vi "SAOMM-OFFSET.vi"(0 "Hexapod VRN":refnum<visa-resource-name>="COM4", 1 "Active Refnum":refnum<vi>, 2 "PrAMS-ACK":refnum<vi>, 7 "output cluster":T1, 13 "MessageType":cluster{string[], u32[]}={["emtError", "emtAreYouThere", "emtAcknowledgment", "emtGetClientType", "emtClientType", "emtGetImageExposureTime", "emtSetImageExposureTime", "emtImageExposureTime", "emtGetOptimalExposureTime", "emtSetOptimalExposureTime", "emtOptimalExposureTime", "emtGetImageEMGain", "emtSetImageEMGain", "emtImageEMGain", "emtGetFPGACtrl", "emtSetFPGACtrl", "emtFPGACtrl", "emtGetImageWidth", "emtSetImageWidth", "emtImageWidth", "emtGetImageHeight", "emtSetImageHeight", "emtImageHeight", "emtGetImageBinning", "emtSetImageBinning", "emtImageBinning", "emtGetImageDisplayFrameRate", "emtSetImageDisplayFrameRate", "emtImageDisplayFrameRate", "emtGetROIWidth", "emtSetROIWidth", "emtROIWidth", "emtGetROIHeight", "emtSetROIHeight", "emtROIHeight", "emtGetROIXOffset", "emtSetROIXOffset", "emtROIXOffset", "emtGetROIYOffset", "emtSetROIYOffset", "emtROIYOffset", "emtStartAcquisition", "mtStopAcquisition", "emtAcquisitionStarted", "emtAcquisitionStopped", "emtGetFalconImage", "emtFalconImage"], [1, 2, 3, 4, 5, 1001, 1101, 1201, 1002, 1102, 1202, 1003, 1103, 1203, 1004, 1104, 1204, 1005, 1105, 1205, 1006, 1106, 1206, 1007, 1107, 1207, 1008, 1108, 1208, 1009, 1109, 1209, 1010, 1110, 1210, 1011, 1111, 1211, 1012, 1112, 1212, 1130, 1131, 1150, 1151, 1070, 1270]}) -> (8 "Error":bool)   [LabVIEW 2019]
uses:
  Polymorphics/Num2littleEndian(DBL).vi
panel:
  out "First Run":bool
  in  "Signature":u32=1886544237
  in  "X":dbl caption="Pos" min=-5.0 max=5.0 format="%.4f"
  in  "Y":dbl caption="Pos" min=-5.0 max=5.0 format="%.4f"
  in  "Z":dbl caption="Pos" min=-5.0 max=5.0 format="%.4f"
  in  "U":dbl caption="Pos" min=-1.0 max=1.0 format="%.4f"
  in  "V":dbl caption="Pos" min=-1.0 max=1.0 format="%.4f"
  # "DÉPLACEMENTS"
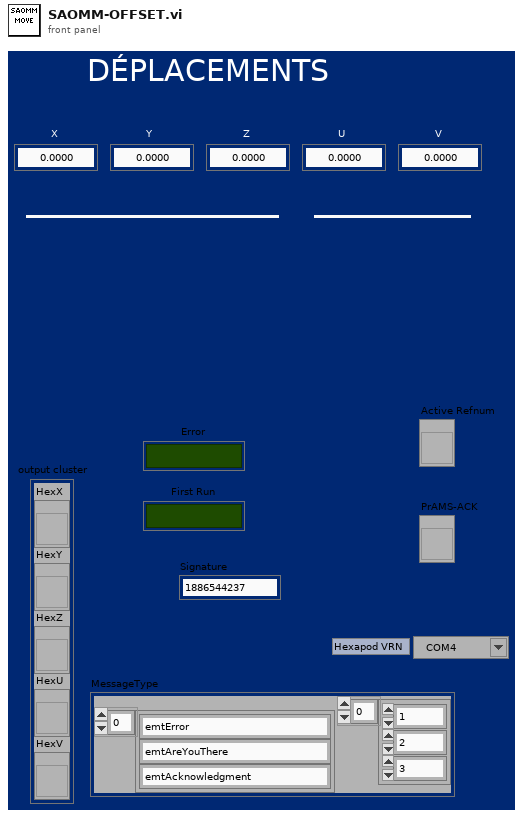
[diagram p1: front panel]
types:
  T1 = cluster{"HexX":refnum<vi>, "HexY":refnum<vi>, "HexZ":refnum<vi>, "HexU":refnum<vi>, "HexV":refnum<vi>}
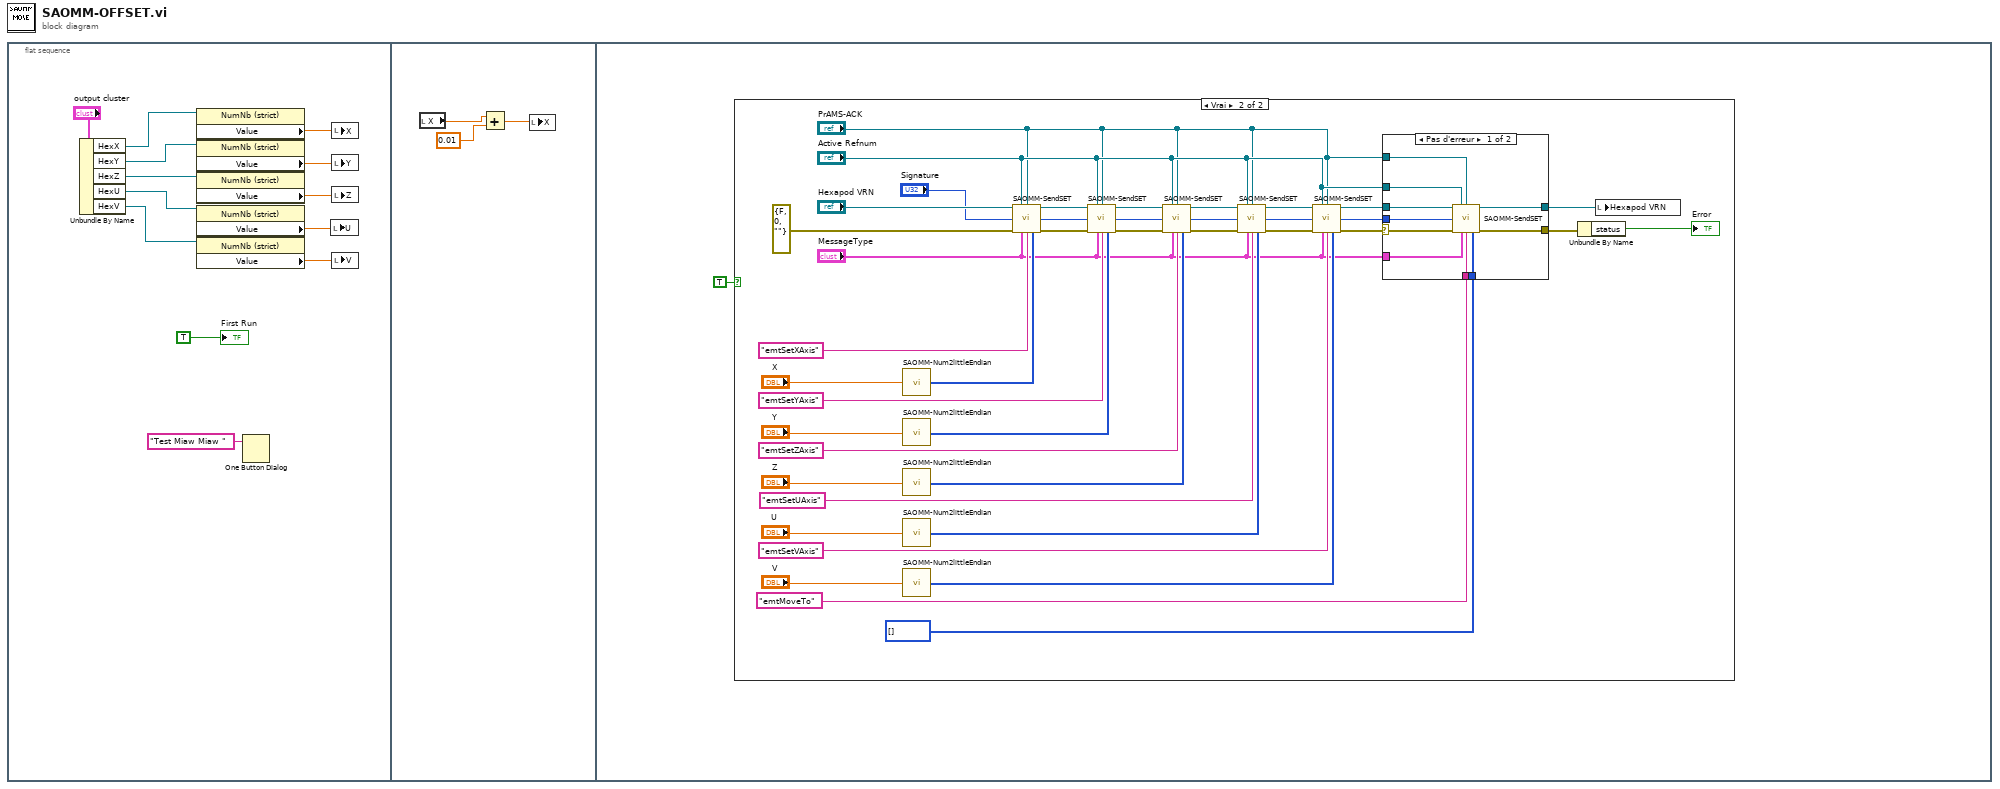
[diagram p0: block diagram]
diagram:
  n1 = flat-sequence {
    frame #0 {
      n2 = Unbundle By Name("output cluster") -> ("HexX"=w11:refnum<vi>, "HexY"=w10:refnum<vi>, "HexZ"=w9:refnum<vi>, "HexU"=w8:refnum<vi>, "HexV"=w7:refnum<vi>)
      n3 = property class="NumNb (strict)"(reference=w11) -> ("Value"=w2:dbl)  [unwired: 1 in, 2 out]
      n4 = property class="NumNb (strict)"(reference=w10) -> ("Value"=w3:dbl)  [unwired: 1 in, 2 out]
      n5 = property class="NumNb (strict)"(reference=w9) -> ("Value"=w4:dbl)  [unwired: 1 in, 2 out]
      n6 = property class="NumNb (strict)"(reference=w8) -> ("Value"=w5:dbl)  [unwired: 1 in, 2 out]
      n7 = property class="NumNb (strict)"(reference=w7) -> ("Value"=w6:dbl)  [unwired: 1 in, 2 out]
      n8 = One Button Dialog(message="Test Miaw Miaw ") -> ()  [unwired: 1 in, 1 out]
      n9 = local write "U"(w5) -> ()
      n10 = local write "X"(w2) -> ()
      n11 = local write "Y"(w3) -> ()
      n12 = local write "Z"(w4) -> ()
      n13 = local write "V"(w6) -> ()
      "First Run" <- TRUE
    }
    frame #1 {
      n14 = local read "X"() -> (w15:dbl)
      n15 = Add(x=w15, y=0.01) -> (x+y=w16:dbl)
      n16 = local write "X"(w16) -> ()
    }
    frame #2 {
      n17 = case shown="Vrai" TRUE {
        frame False {
        }
        frame True {
          n18 = call-poly "SAOMM-Num2littleEndian.vi"("Number"="X") -> ("LiitleEndianedData"=w40:u8[])  [unwired: 14 in]
          n19 = call-poly "SAOMM-Num2littleEndian.vi"("Number"="Y") -> ("LiitleEndianedData"=w41:u8[])  [unwired: 14 in]
          n20 = call-poly "SAOMM-Num2littleEndian.vi"("Number"="Z") -> ("LiitleEndianedData"=w42:u8[])  [unwired: 14 in]
          n21 = call-poly "SAOMM-Num2littleEndian.vi"("Number"="U") -> ("LiitleEndianedData"=w45:u8[])  [unwired: 14 in]
          n22 = call-poly "SAOMM-Num2littleEndian.vi"("Number"="V") -> ("LiitleEndianedData"=w46:u8[])  [unwired: 14 in]
          n23 = call "SAOMM-SendSET.vi"("PRAMMS-COMM IN"="Hexapod VRN", "Active Refnum"="Active Refnum", "PrAMS-ACK"="PrAMS-ACK", "Signature"="Signature", "Error IN"=errorcluster {"status"=FALSE, "code"=0, "source"=""}, "MessageType"="MessageType", "Active SET"="emtSetXAxis", "Value (little endianed byte array)"=w40) -> ("PRAMMS-COMM OUT"=w31:refnum<visa-resource-name>, "Error OUT"=w37:errorcluster)  [unwired: 4 in, 2 out]
          n24 = call "SAOMM-SendSET.vi"("PRAMMS-COMM IN"=w31, "Active Refnum"="Active Refnum", "PrAMS-ACK"="PrAMS-ACK", "Signature"="Signature", "Error IN"=w37, "MessageType"="MessageType", "Active SET"="emtSetYAxis", "Value (little endianed byte array)"=w41) -> ("PRAMMS-COMM OUT"=w32:refnum<visa-resource-name>, "Error OUT"=w36:errorcluster)  [unwired: 4 in, 2 out]
          n25 = call "SAOMM-SendSET.vi"("PRAMMS-COMM IN"=w32, "Active Refnum"="Active Refnum", "PrAMS-ACK"="PrAMS-ACK", "Signature"="Signature", "Error IN"=w36, "MessageType"="MessageType", "Active SET"="emtSetZAxis", "Value (little endianed byte array)"=w42) -> ("PRAMMS-COMM OUT"=w52:refnum<visa-resource-name>, "Error OUT"=w35:errorcluster)  [unwired: 4 in, 2 out]
          n26 = call "SAOMM-SendSET.vi"("PRAMMS-COMM IN"=w52, "Active Refnum"="Active Refnum", "PrAMS-ACK"="PrAMS-ACK", "Signature"="Signature", "Error IN"=w35, "MessageType"="MessageType", "Active SET"="emtSetUAxis", "Value (little endianed byte array)"=w45) -> ("PRAMMS-COMM OUT"=w53:refnum<visa-resource-name>, "Error OUT"=w34:errorcluster)  [unwired: 4 in, 2 out]
          n27 = call "SAOMM-SendSET.vi"("PRAMMS-COMM IN"=w53, "Active Refnum"="Active Refnum", "PrAMS-ACK"="PrAMS-ACK", "Signature"="Signature", "Error IN"=w34, "MessageType"="MessageType", "Active SET"="emtSetVAxis", "Value (little endianed byte array)"=w46) -> ("PRAMMS-COMM OUT"=w51:refnum<visa-resource-name>, "Error OUT"=w50:errorcluster)  [unwired: 4 in, 2 out]
          n28 = case shown="Pas d'erreur" w50 {
            selector: w50 -> [w55 w64]
            tunnel: "Active Refnum" -> [w63 _]
            tunnel: "PrAMS-ACK" -> [w62 _]
            tunnel: "Signature" -> [w61 _]
            tunnel: [w60 w65] -> w33
            tunnel: [w59 w64] -> w19
            tunnel: "MessageType" -> [w58 _]
            tunnel: "emtMoveTo" -> [w57 _]
            tunnel: u8[] [] ("Value (little endianed byte array)") -> [w56 _]
            tunnel: w51 -> [w54 w65]
            frame No Error {
              n29 = call "SAOMM-SendSET.vi"("PRAMMS-COMM IN"=w54, "Active Refnum"=w63, "PrAMS-ACK"=w62, "Signature"=w61, "Error IN"=w55, "MessageType"=w58, "Active SET"=w57, "Value (little endianed byte array)"=w56) -> ("PRAMMS-COMM OUT"=w60:refnum<visa-resource-name>, "Error OUT"=w59:errorcluster)  [unwired: 4 in, 2 out]
            }
            frame Error {
            }
          }
          n30 = Unbundle By Name(w19) -> ("status"=→"Error":bool)
          n31 = local write "Hexapod VRN"(w33) -> ()
        }
      }
    }
  }
